vi "Start Up File.vi"(2 "error in (no error)":errorcluster, 3 "FileName":string="Config") -> (0 "error out":errorcluster, 1 "FilePath":path)   [LabVIEW 2018]
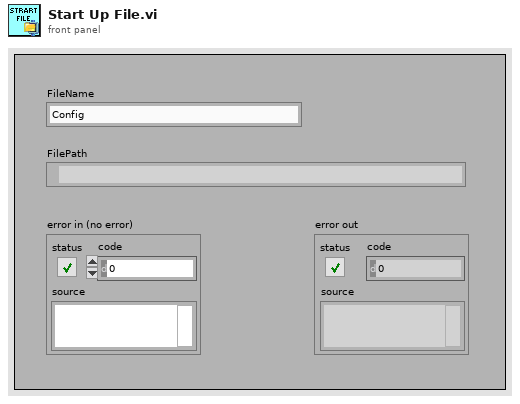
[diagram p1: front panel]
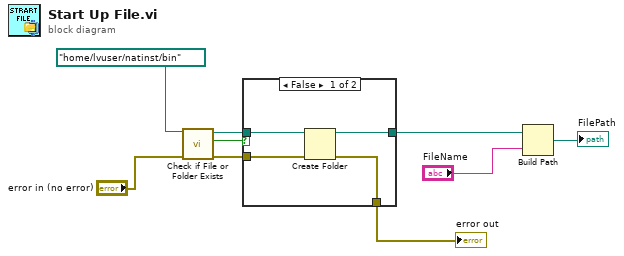
[diagram p0: block diagram]
diagram:
  n1 = call <vilib>:"Check if File or Folder Exists.vi"("error in (no error)"="error in (no error)", "path"=path "/home/lvuser/natinst/bin") -> ("error out"=w4:errorcluster, "file or folder exists?"=w8:bool, "dup path"=w7:path)  [unwired: 7 in]
  n2 = case shown="False" w8 {
    tunnel: w7 -> [w13 w15]
    tunnel: [w12 w15] -> w6
    tunnel: w4 -> [w11 w14]
    tunnel: [w10 w14] -> w2
    frame False {
      n3 = Create Folder(path (use dialog)=w13, error in=w11) -> (created path=w12:path, error out=w10:errorcluster)  [unwired: 1 in, 1 out]
    }
    frame True {
    }
  }
  "error out" <- w2
  n4 = Build Path(base path=w6, name or relative path="FileName") -> (appended path=→"FilePath":path)
